vi "StringSplitIntoThree.vi"(9 "Max word length":i32=5, 11 "String":string) -> (1 "Line 3":string, 2 "Line 2":string, 3 "Line 1":string)   [LabVIEW 2019, in "gRPC Template Creation Utility.lvlib"]
uses:
  gRPC Template Creation Utility.lvlib
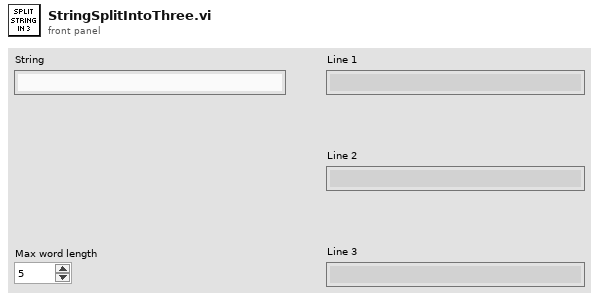
[diagram p1: front panel]
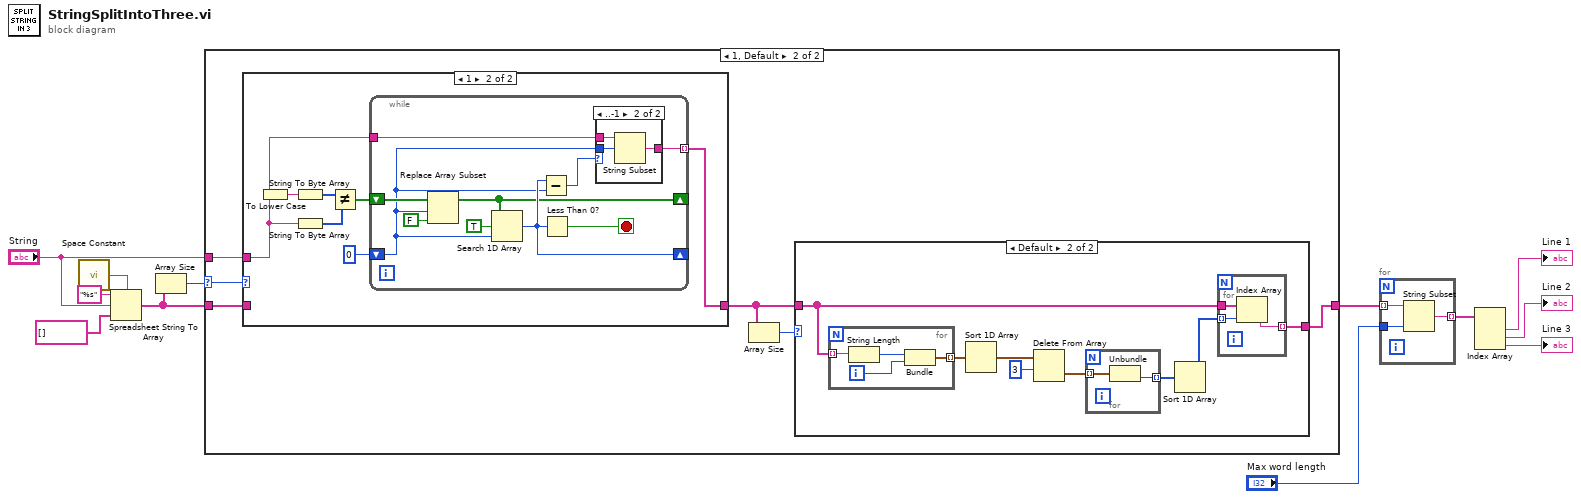
[diagram p0: block diagram]
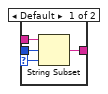
[diagram p4: hidden frame]
diagram:
  n1 = call <vilib>:"Space Constant.vi"() -> ("String"=w11:string)
  n2 = Spreadsheet String To Array(delimiter (Tab)=w11, format string="%s", spreadsheet string="String", array type (2D Dbl)=string[] []) -> (array=w8:string[])
  n3 = Array Size(array=w8) -> (size(s)=w9:i32)
  n4 = case shown="1, Default" w9 {
    selector: w9 -> [_ w18]
    tunnel: w8 -> [w13 w17]
    tunnel: "String" -> [_ w19]
    tunnel: [w13 w14] -> w3
    frame 2, 3 {
    }
    frame 1, Default {
      n5 = case shown="1" w18 {
        tunnel: w19 -> [_ w24]
        tunnel: [w20 w22] -> w16
        tunnel: w17 -> [w20 _]
        frame Default {
        }
        frame 1 {
          n6 = To Lower Case(string=w24) -> (all lower case string=w27:string)
          n7 = String To Byte Array(string=w27) -> (unsigned byte array=w26:u8[])
          n8 = String To Byte Array(string=w24) -> (unsigned byte array=w25:u8[])
          n9 = Not Equal?(x=w26, y=w25) -> (x != y?=w21:bool[])
          n10 = while {
            tunnel: w24 -> [w36]
            shift-right: [w33] -> _
            shift-left: 0 ("start index (0)") -> [w29]
            tunnel: [w35] -> w22 mode=indexing
            shift-right: [w30] -> _
            shift-left: w21 -> [w31]
            stop <- w34 stop-if-true
            n11 = Replace Array Subset(array=w31, new element=FALSE ("new element/subarray"), index=w29) -> (w30:bool[])
            n12 = Search 1D Array(1D array=w30, element=TRUE, start index (0)=w29) -> (index of element=w33:i32)
            n13 = Subtract(x=w33, y=w29) -> (x-y=w28:i32)
            n14 = Less Than 0?(x=w33) -> (x < 0?=w34:bool)
            n15 = case shown="..-1" w28 {
              selector: w28 -> [w38 _]
              tunnel: w36 -> [w41 w44]
              tunnel: [w40 w43] -> w35
              tunnel: w29 -> [w39 w42]
              frame Default {
                n16 = String Subset(string=w41, offset (0)=w39, length (rest)=w38) -> (substring=w40:string)
              }
              frame ..-1 {
                n17 = String Subset(string=w44, offset (0)=w42) -> (substring=w43:string)  [unwired: 1 in]
              }
            }
          }
        }
      }
      n18 = Array Size(array=w16) -> (size(s)=w15:i32)
      n19 = case shown="Default" w15 {
        tunnel: w16 -> [w45 w48]
        tunnel: [w45 w46] -> w14
        frame 1 {
        }
        frame Default {
          n20 = for {
            tunnel: w48 -> [w62] mode=indexing
            tunnel: [w59] -> w53 mode=indexing
            i -> [w60]
            n21 = String Length(string=w62) -> (length=w61:i32)
            n22 = Bundle(w61, w60) -> (w59:cluster{i32, i32})  [unwired: 1 in]
          }
          n23 = Sort 1D Array(array=w53) -> (sorted array=w49:cluster{i32, i32}[])
          n24 = Delete From Array(array=w49, length=3) -> (deleted portion=w51:cluster{i32, i32}[])  [unwired: 1 in, 1 out]
          n25 = for {
            tunnel: w51 -> [w58] mode=indexing
            tunnel: [w57] -> w50 mode=indexing
            n26 = Unbundle(w58) -> (w57:i32)  [unwired: 1 out]
          }
          n27 = Sort 1D Array(array=w50) -> (sorted array=w47:i32[])
          n28 = for {
            tunnel: w48 -> [w56]
            tunnel: w47 -> [w55] mode=indexing
            tunnel: [w54] -> w46 mode=indexing
            n29 = Index Array(array=w56, index=w55) -> (element=w54:string)
          }
        }
      }
    }
  }
  n30 = for {
    tunnel: w3 -> [w65] mode=indexing
    tunnel: "Max word length" -> [w64]
    tunnel: [w63] -> w1 mode=indexing
    n31 = String Subset(string=w65, length (rest)=w64) -> (substring=w63:string)  [unwired: 1 in]
  }
  n32 = Index Array(array=w1) -> (element #1=→"Line 1":string, element #2=→"Line 2":string, element #3=→"Line 3":string)  [unwired: 3 in]
